vi "Read Error Mode.vi"(8 "error in (no error)":errorcluster, 11 "gScript Interpreter in":refnum<class "gScript Interpreter.lvclass">) -> (0 "error out":errorcluster, 2 "Error Mode":T1, 3 "gScript Interpreter out":refnum<class "gScript Interpreter.lvclass">)   [LabVIEW 2023, in "gScript Interpreter.lvclass"]
uses:
  gScript Interpreter.lvclass
  Type Definitions/Error Mode.ctl
  gScript Interpreter.lvclass/gScript Interpreter.ctl
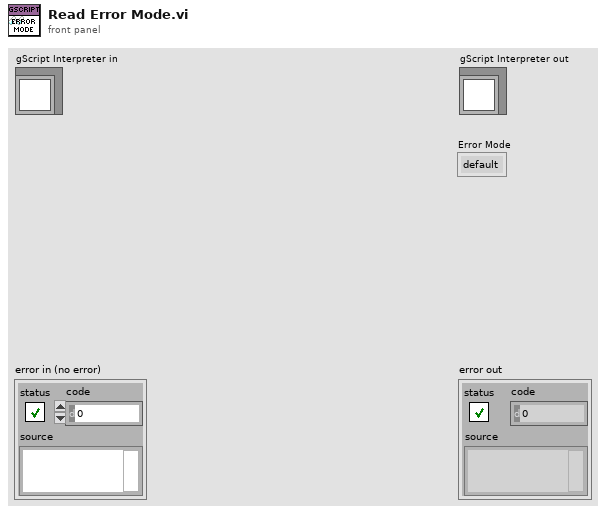
[diagram p1: front panel]
types:
  T1 = typedef "Error Mode.ctl" = enum16{"default", "prompt", "setvar"}
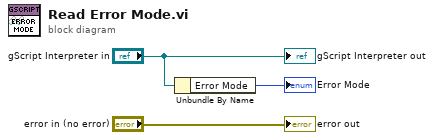
[diagram p0: block diagram]
diagram:
  n1 = Unbundle By Name("gScript Interpreter in") -> ("Error Mode"=→"Error Mode":T1)
  "error out" <- "error in (no error)"
  "gScript Interpreter out" <- "gScript Interpreter in"
